vi "Arm Controller.vi"(8 "error in":errorcluster) -> ()   [LabVIEW 2018]
doc: "This VI executes continuously carrying out the current operation and responding to updates or new operations. It will often contain the timing or control code that is difficult to place directly in TeleOp. This VI generally opens all sensors and motors and isolates the rest of the robot code from knowing how the operations are carried out."
uses:
  <vilib>/Rock Robotics/WPI/Framework/Completion Status.ctl
  Arm Setpoints.ctl
  Arm Operations.ctl
  Arm Positions.ctl
  <vilib>/Rock Robotics/WPI/ThirdParty/Phoenix-LabVIEW/Motor Controller/Controls/CTRE_Phoenix_MotorControl_LimitSwitchSource_Local.ctl
  <vilib>/Rock Robotics/WPI/ThirdParty/Phoenix-LabVIEW/Motor Controller/Controls/CTRE_Phoenix_MotorControl_LimitSwitchNormal.ctl
  <vilib>/Rock Robotics/WPI/ThirdParty/Phoenix-LabVIEW/Motor Controller/Controls/CTRE_Phoenix_MotorControl_FeedbackDevice.ctl
  Turret Position.ctl
  <vilib>/Rock Robotics/WPI/ThirdParty/Phoenix-LabVIEW/Motor Controller/Controls/CTRE_Phoenix_MotorControl_ControlMode.ctl
  <vilib>/Rock Robotics/WPI/ThirdParty/Phoenix-LabVIEW/Motor Controller/Get/CTRE_Phoenix_MotorController_GetOutputCurrent_Enhanced.vi
  <vilib>/Rock Robotics/WPI/ThirdParty/Phoenix-LabVIEW/Motor Controller/Get/CTRE_Phoenix_MotorController_GetLimitSwitchStates.vi
  Arm Published Globals.vi
  Arm Constants.vi
  <vilib>/Rock Robotics/WPI/ThirdParty/Phoenix-LabVIEW/Motor Controller/Get/CTRE_Phoenix_MotorController_GetSelectedSensorData.vi
  <vilib>/Rock Robotics/Network Tables/NT Write Number.vi
  <vilib>/ptbypt/NI_PtbyPt.lvlib
  <vilib>/Rock Robotics/WPI/ThirdParty/Phoenix-LabVIEW/Controls/CTRE_Phoenix_Params.ctl
  <vilib>/Rock Robotics/Network Tables/NT Write Boolean.vi
panel:
  in  "P @ parallel to gnd elbow":dbl
  in  "P @ parallel to gnd":dbl
  in  "New Sensor Position 2":i32=-2
  in  "New Sensor Position":i32=-241
  in  "x":i32=500
  out "extensionLength":dbl=30.50305897767295
  out "wrist angle(deg)":dbl=27.45141836050927
  out "shoulder angle(deg)":dbl=92.24007561436673
  out "turret angle(deg)":dbl=45.049846153846154
  out "Theta4":dbl=207.45141836050928
  out "Theta3":dbl=36.40857303428192
  out "elbow angle(deg)":dbl=-51.35135135135135
  out "Position - Encoder Counts":T1(graph)={"Position (Raw Sensor Units)"=8134, "Position (Raw Sensor Units)"=-2127, "Position (Raw Sensor Units)"=-2299, "Position (Raw Sensor Units)"=1229}
  out "Position - Degrees":T2(graph)={"turret angle(deg)"=45.049846153846154, "shoulder angle(deg)"=92.24007561436673, "elbow angle(deg)"=-51.35135135135135, "wrist angle(deg)"=27.45141836050927}
  in  "Disable Logging":bool
  out "Current":T3(graph)
  in  "Interactive Values":T4
  out "Current\nCmd":string="Started at  22:56:16.335\nDefault: Reserve,  S 0.0, D 0.000000"
  in  "Buttons":cluster{"Execute Cmd":bool, "Abort Cmd":bool}
  out "Command Timing":cluster{"Start Time (ms)":u32, "Iterations":i32}={"Start Time (ms)"=8369965, "Iterations"=0}
  out "Status":T7
  # "Interactive Command: You may fill in the settings for a command\nand schedule it with the Execute button. You can observe and abort\nany command while fine tuning the code for the controller."
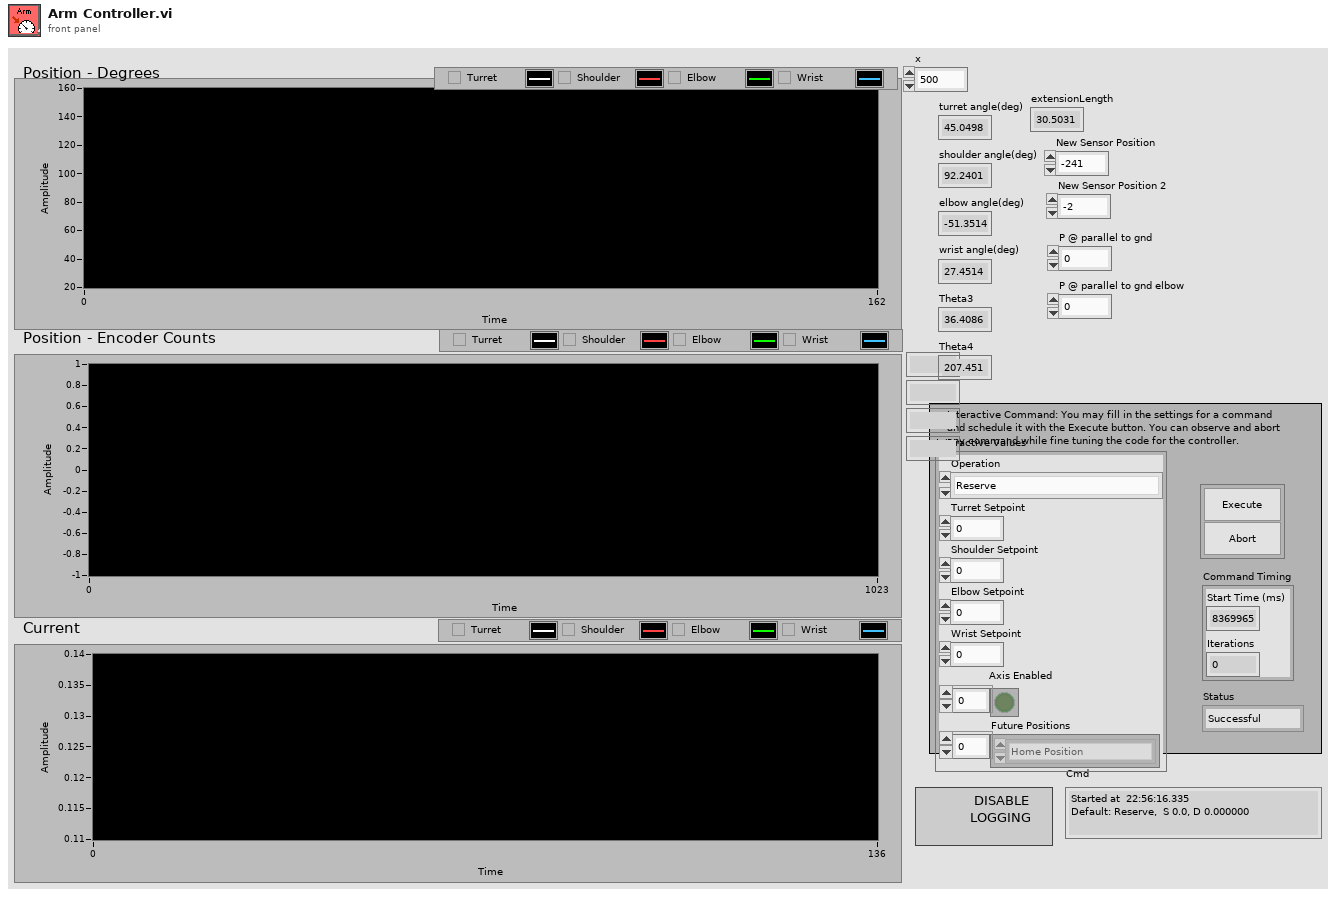
[diagram p1: front panel]
types:
  T1 = cluster{"Position (Raw Sensor Units)":i32, "Position (Raw Sensor Units)":i32, "Position (Raw Sensor Units)":i32, "Position (Raw Sensor Units)":i32}
  T2 = cluster{"turret angle(deg)":dbl, "shoulder angle(deg)":dbl, "elbow angle(deg)":dbl, "wrist angle(deg)":dbl}
  T3 = cluster{"Output Current":dbl, "Output Current":dbl, "Output Current":dbl, "Output Current":dbl}
  T4 = typedef "Arm Setpoints.ctl" = cluster{"Operation":T5, "Turret Setpoint":dbl, "Shoulder Setpoint":dbl, "Elbow Setpoint":dbl, "Wrist Setpoint":dbl, "Axis Enabled":bool[], "Future Positions":T6[]}
  T5 = typedef "Arm Operations.ctl" = enum16{"Reserve", "Read Current", "Immediate", "Move arm to position", "Reset Encoders", "Reset Turret", "Reset Shoulder", "Reset Elbow", "Reset Wrist", "Hold Encoder Counts"}
  T6 = typedef "Arm Positions.ctl" = enum16{"Home Position", "Safe Position", "Hatch - Ground", "Hatch - Low", "Hatch - Middle", "High - Safe", "Hatch - High", "Cargo - Low", "Cargo - Middle", "Cargo - High", "Cargo - Loading Station", "Hatch - Loading Station", "Cargo - Ground", "Turret - Left", "Turret - Front", "Turret - Right", "Turret - Back", "Climbing - Forward", "Middle - Safe", "Low - Safe", "Safe Elbow up"}
  T7 = typedef "Completion Status.ctl" = enum16{"Successful", "Aborted", "Incomplete"}
  T8 = typedef "CTRE_Phoenix_MotorControl_FeedbackDevice.ctl" = i8
  T9 = typedef "CTRE_Phoenix_MotorControl_LimitSwitchNormal.ctl" = enum16{"Normally Open", "Normally Closed", "Disabled"}
  T10 = typedef "CTRE_Phoenix_MotorControl_LimitSwitchSource_Local.ctl" = enum16{"Feedback Connector", "Remote Talon SRX", "Remote CANifier", "Deactivated"}
  T11 = typedef "CTRE_Phoenix_Params.ctl" = u16
  T12 = typedef "WPI_MotorControlDeviceRef.ctl" = cluster{"DeviceStatus":errorcluster, "Type":T13, "PWM":cluster{"PWM Channel":T14, "DeadBand":T15}, "CAN":cluster{"Device Number":u8, "SetOutput VI Ref":variant, "GetOutput VI Ref":variant, "Enable VI Ref":variant, "Disable VI Ref":variant, "Data":variant}, "Invert":bool, "DIO PWM":cluster{"PWM \"Enable\" Channel":T14, "DIOChannel":T16, "PWM Rate":dbl}}
  T13 = typedef "WPI_MotorControlType.ctl" = enum16{"PWM", "CAN", "DIO PWM"}
  T14 = typedef "FPGA_DIOPWMChannel.ctl" = enum8{"PWM 0", "PWM 1", "PWM 2", "PWM 3", "PWM 4", "PWM 5", "PWM 6", "PWM 7", "PWM 8", "PWM 9", "PWM MXP 0", "PWM MXP 1", "PWM MXP 2", "PWM MXP 3", "PWM MXP 4", "PWM MXP 5", "PWM MXP 6", "PWM MXP 7", "PWM MXP 8", "PWM MXP 9", "Invalid"}
  T15 = typedef "WPI_PWMDeadband.ctl" = cluster{"Name":string, "maxPositivePwm":i32, "minPositivePwm":i32, "centerPwm":i32, "maxNegativePwm":i32, "minNegativePwm":i32, "angularRange":u16}
  T16 = typedef "FPGA_DIOChannel.ctl" = enum8{"DIO 0", "DIO 1", "DIO 2", "DIO 3", "DIO 4", "DIO 5", "DIO 6", "DIO 7", "DIO 8", "DIO 9", "DIO MXP 0", "DIO MXP 1", "DIO MXP 2", "DIO MXP 3", "DIO MXP 4", "DIO MXP 5", "DIO MXP 6", "DIO MXP 7", "DIO MXP 8", "DIO MXP 9", "DIO MXP 10", "DIO MXP 11", "DIO MXP 12", "DIO MXP 13", "DIO MXP 14", "DIO MXP 15", "SPI Port CS1", "SPI Port CS2", "SPI Port CS3", "SPI Port MISO", "SPI Port MOSI", "Invalid"}
  T17 = typedef "Command Status Info.ctl" = cluster{"Name":string, "Status":T7, "notifier out":T18}
  T18 = typedef "Completion Notifier.ctl" = refnum<notifier>
  T19 = cluster{"Current Command":T4, "Command Timing":cluster{"Start Time (ms)":u32, "Iterations":i32}, "Command Arguments":cluster{"Command Info":T17, "Description":string, "Default Command":T4, "queue out":refnum<queue>, "Subsystem Name":string}}
  T20 = typedef "Turret Position.ctl" = enum16{"Back", "Left", "Front", "Right"}
  T21 = cluster{"Position (Raw Sensor Units)":i32, "Position (Raw Sensor Units)":i32, i32, i32}
  T22 = typedef "CTRE_Phoenix_MotorControl_ControlMode.ctl" = u16
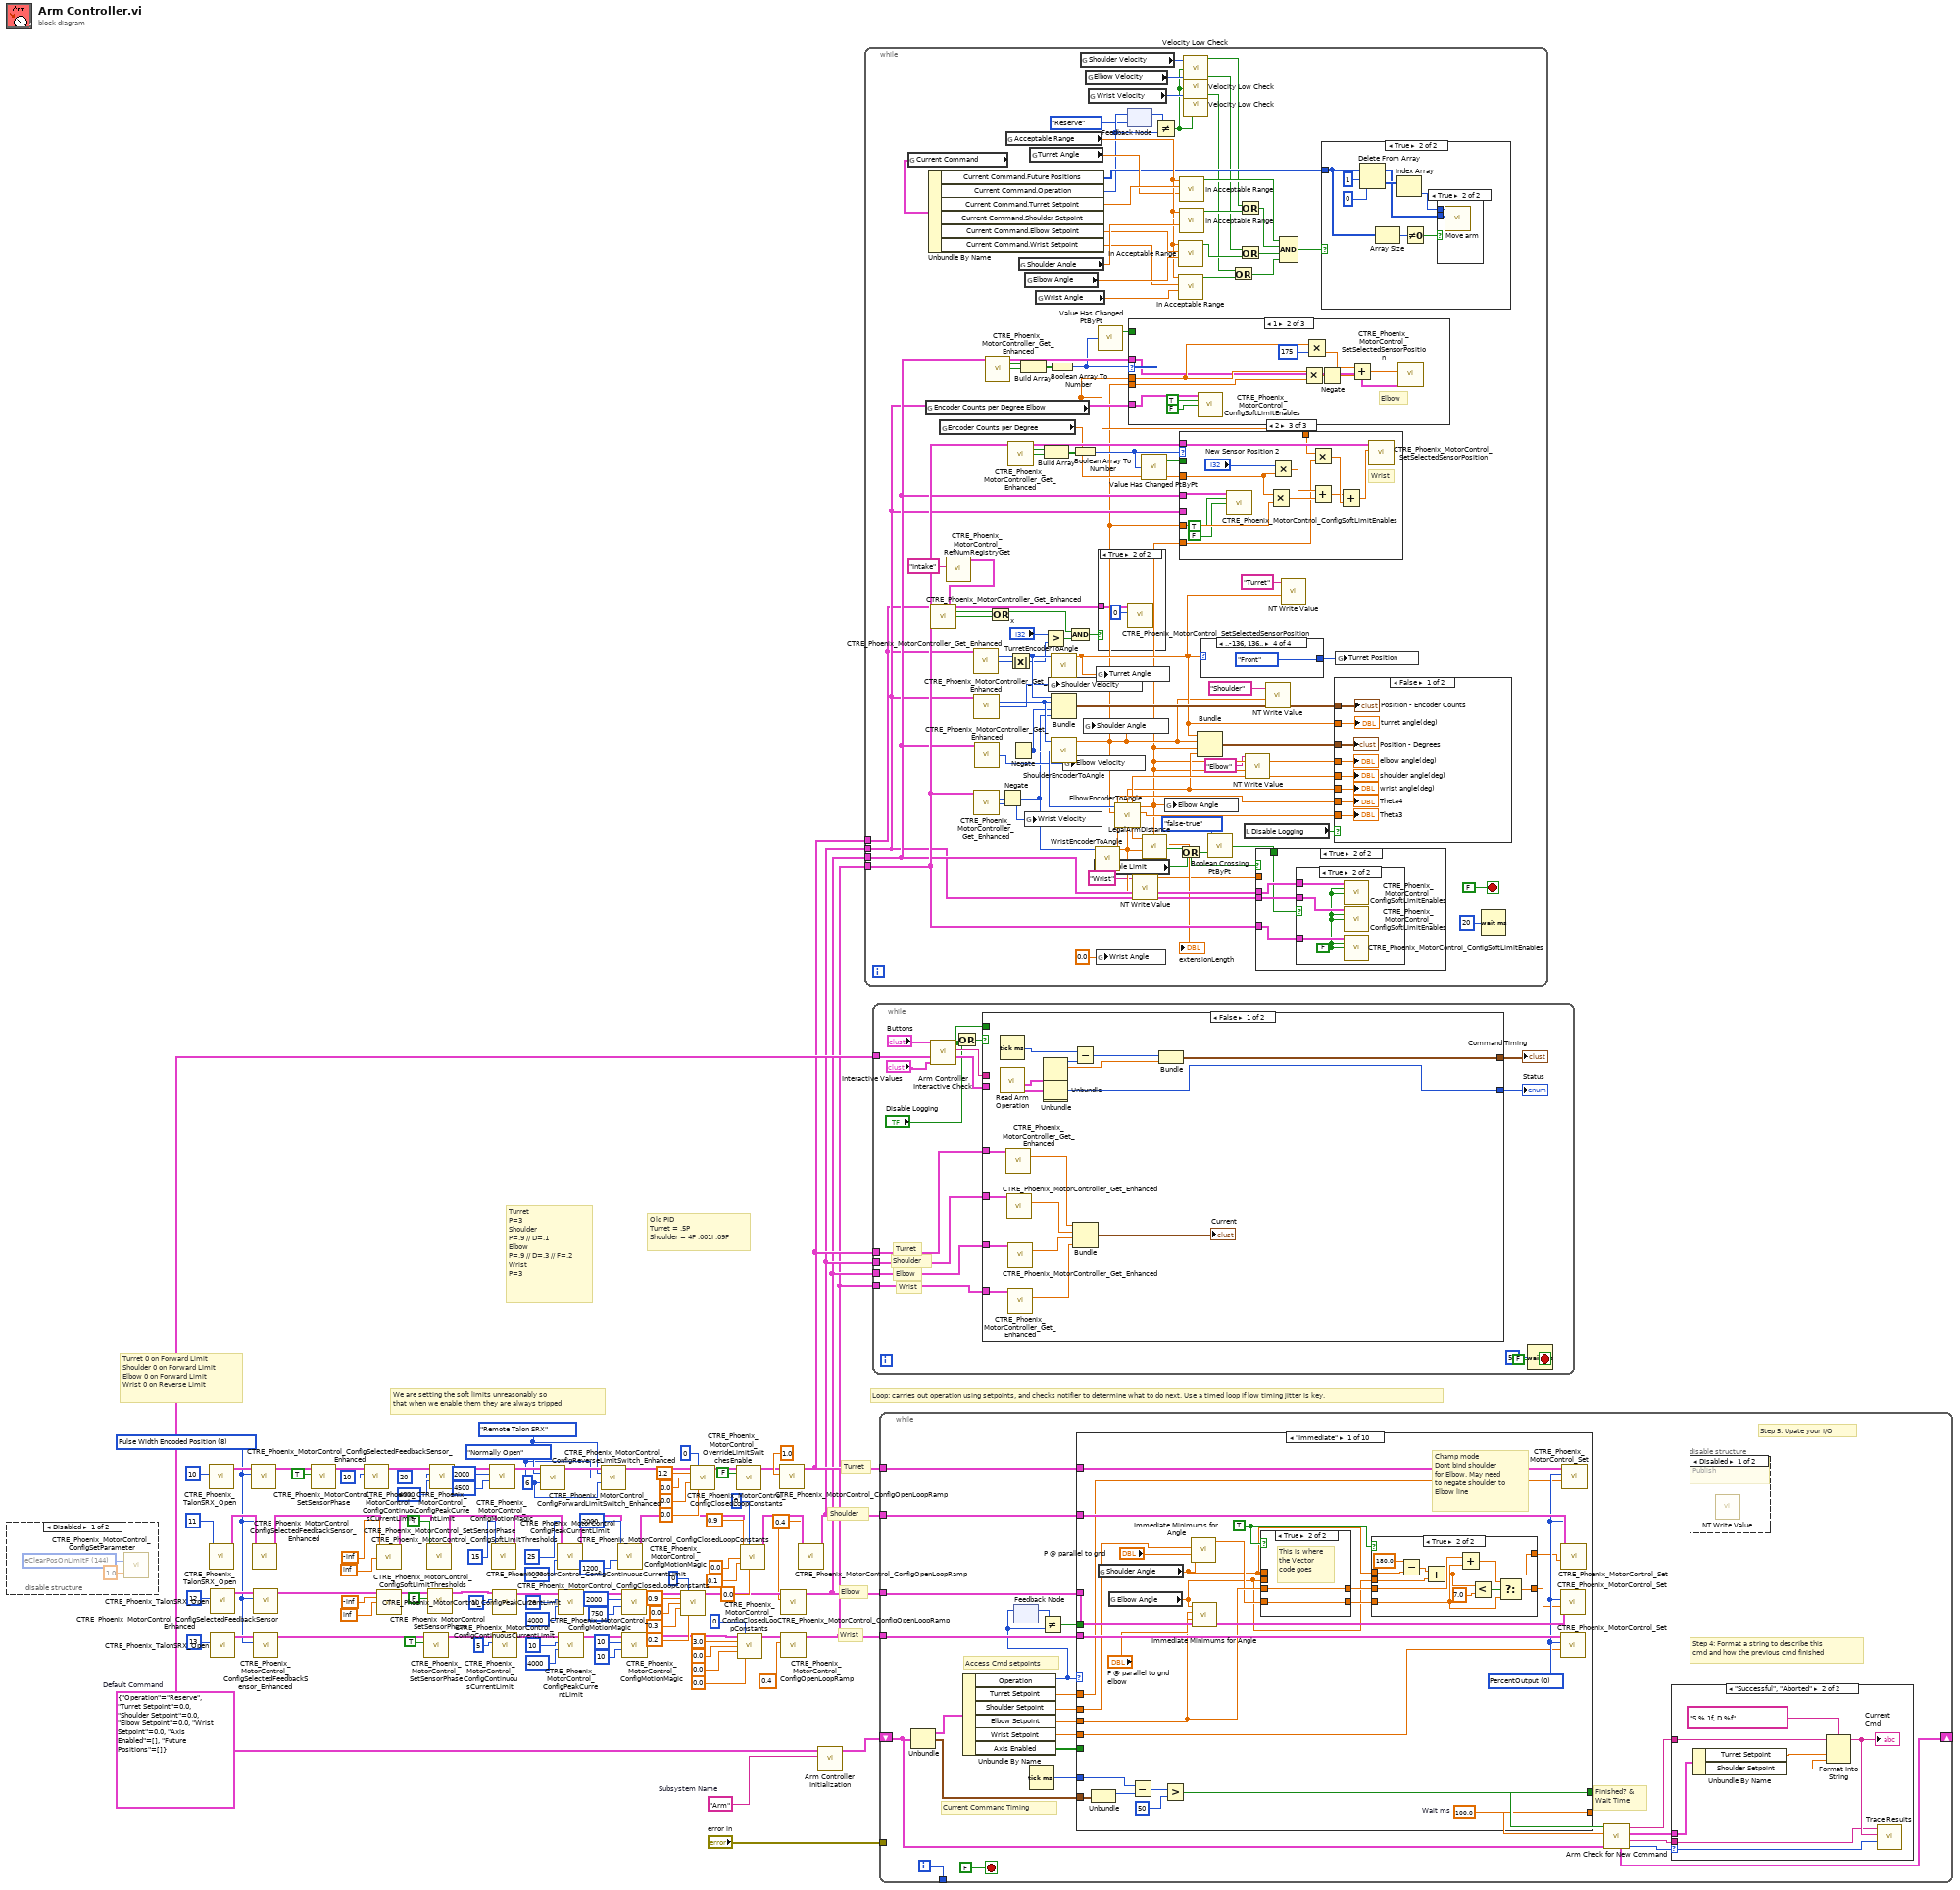
[diagram p0: block diagram]
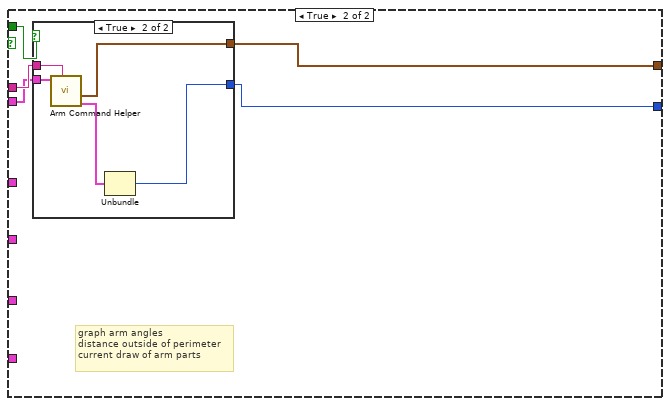
[diagram p3: hidden frame]
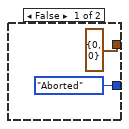
[diagram p4: hidden frame]
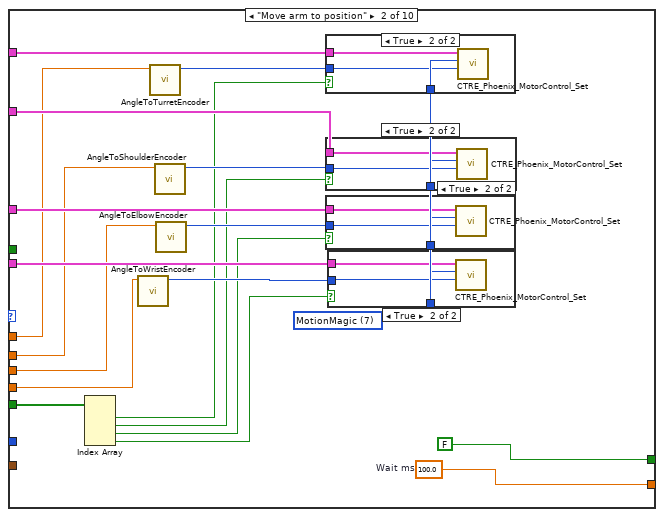
[diagram p9: hidden frame]
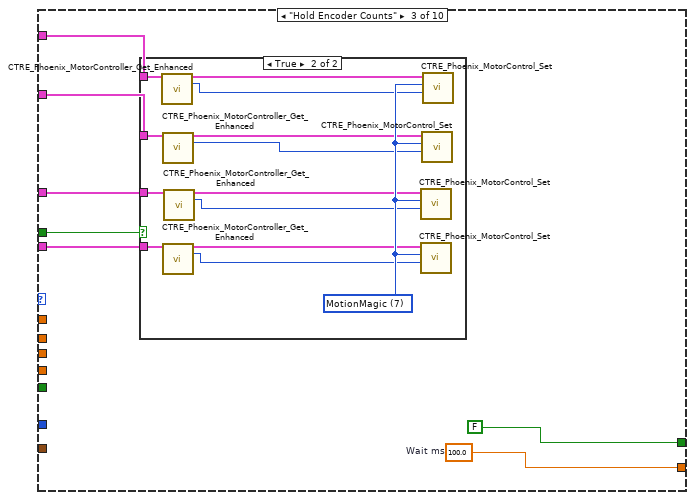
[diagram p14: hidden frame]
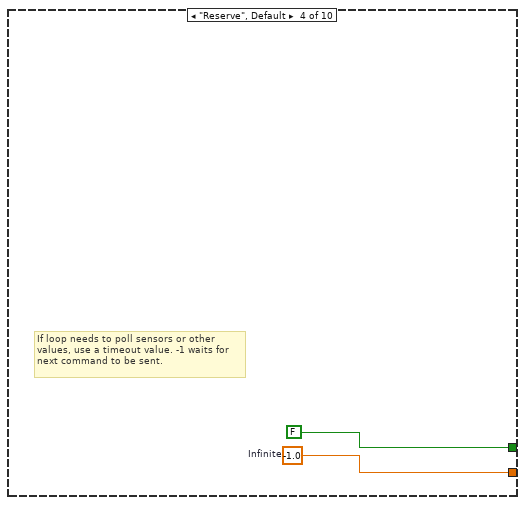
[diagram p16: hidden frame]
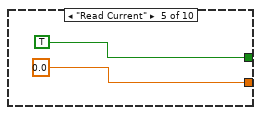
[diagram p17: hidden frame]
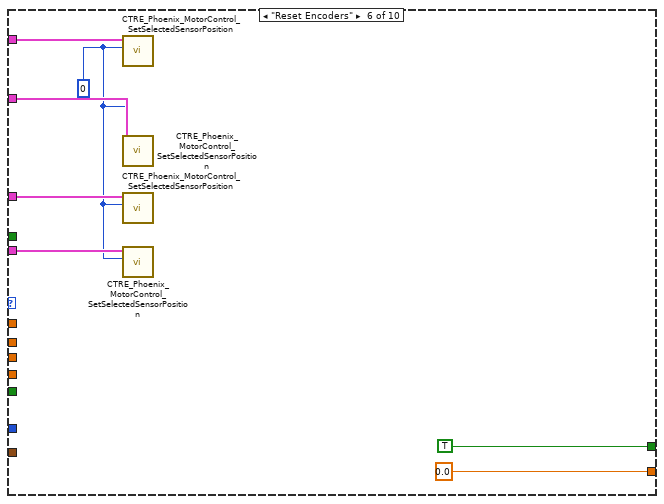
[diagram p18: hidden frame]
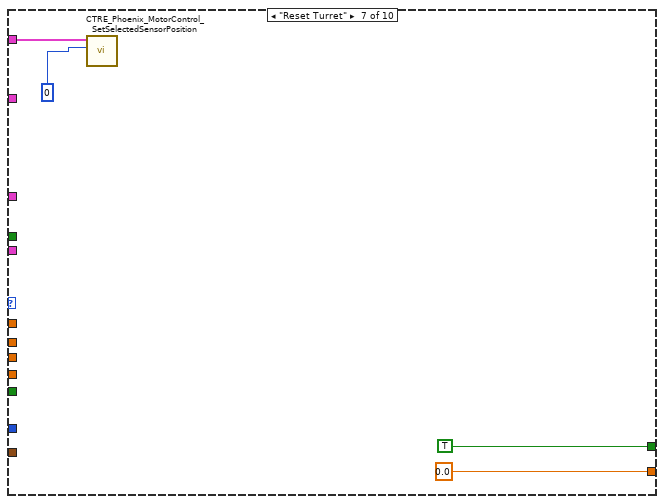
[diagram p19: hidden frame]
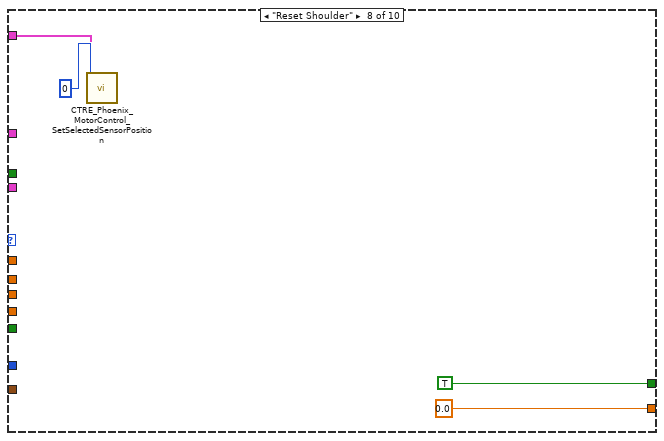
[diagram p20: hidden frame]
diagram:
  w2 = 0.4 ("secondsFromNeutralToFull")
  w3 = T8 8 items=["QuadEncoder"=0, "Analog"=2, "Tachometer"=4, "Pulse Width Encoded Position"=8, "Sensor Sum (S0 + S1)"=9, "Sensor Difference (D0 - D1)"=10, "Remote Source 0"=11, "Remote Source 1"=12, "Software Emulated"=15] ("Feedback Device")
  w37 = CTRE_Phoenix_MotorControl_LimitSwitchNormal."Normally Open" ("NormallyOpenOrClosed")
  w36 = 6 ("deviceID")
  w38 = CTRE_Phoenix_MotorControl_LimitSwitchSource_Local."Remote Talon SRX" ("Limit Switch Source")
  w98 = T4 {"Operation"=enum."Reserve", "Turret Setpoint"=0.0, "Shoulder Setpoint"=0.0, "Elbow Setpoint"=0.0, "Wrist Setpoint"=0.0, "Axis Enabled"=[], "Future Positions"=[]}  # Default Command
  w99 = "Arm"  # Subsystem Name
  # "We are setting the soft limits unreasonably so\nthat when we enable them they are always tripped"
  # "Turret 0 on Forward Limit\nShoulder 0 on Forward Limit\nElbow 0 on Forward Limit\nWrist 0 on Reverse Limit"
  # "Old PID\nTurret = .5P\nShoulder = 4P .001I .09F"
  # "Turret\nP=3\nShoulder\nP=.9 // D=.1\nElbow\nP=.9 // D=.3 // F=.2\nWrist\nP=3"
  # "Wrist"
  # "Elbow"
  # "Shoulder"
  # "Turret"
  # "Loop: carries out operation using setpoints, and checks notifier to determine what to do next. Use a timed loop if low timing jitter is key."
  n1 = disable-structure shown="Disabled" {
    frame Disabled {
      w103 = T11 144 items=["eOnBoot_BrakeMode"=31, "eQuadFilterEn"=91, "eQuadIdxPolarity"=108, "eClearPositionOnIdx"=100, "eMotionProfileHasUnderrunErr"=119, "eMotionProfileTrajectoryPointDurationMs"=120, "eClearPosOnLimitF"=144, "eClearPosOnLimitR"=145, "eStatusFramePeriod"=300, "eOpenLoopRamp"=301, "eClosedLoopRamp"=302, "eNeutralDeadband"=303, "ePeakPosOutput"=305, "eNominalPosOutput"=306, "ePeakNegOutput"=307, "eNominalNegOutput"=308, "eProfileParamSlot_P"=310, "eProfileParamSlot_I"=311, "eProfileParamSlot_D"=312, "eProfileParamSlot_F"=313, "eProfileParamSlot_IZone"=314, "eProfileParamSlot_AllowableErr"=315, "eProfileParamSlot_MaxIAccum"=316, "eProfileParamSlot_PeakOutput"=317, "eClearPositionOnLimitF"=320, "eClearPositionOnLimitR"=321, "eClearPositionOnQuadIdx"=322, "eSampleVelocityPeriod"=325, "eSampleVelocityWindow"=326, "eFeedbackSensorType"=330, "eSelectedSensorPosition"=331, "eFeedbackNotContinuous"=332, "eRemoteSensorSource"=333, "eRemoteSensorDeviceID"=334, "eSensorTerm"=335, "eRemoteSensorClosedLoopDisableNeutralOnLOS"=336, "ePIDLoopPolarity"=337, "ePIDLoopPeriod"=338, "eSelectedSensorCoefficient"=339, "eForwardSoftLimitThreshold"=340, "eReverseSoftLimitThreshold"=341, "eForwardSoftLimitEnable"=342, "eReverseSoftLimitEnable"=343, "eNominalBatteryVoltage"=350, "eBatterVoltageFilterSize"=351, "eContinuousCurrentLimitAmps"=360, "eContinuousCurrentLimitMs"=361, "ePeakCurrentLimitAmps"=362, "eClosedLoopIAccum"=370, "eCustomParam"=380, "eStickyFaults"=390, "eAnalogPosition"=400, "eQuadraturePosition"=401, "ePulseWidthPosition"=402, "eMotMag_Accel"=410, "eMotMag_VelCruise"=411, "eLimitSwitchSource"=421, "eLimitSwitchNormClosedAndDis"=422, "eLimitSwitchDisabledNeutralOnLOS"=423, "eLimitSwitchRemoteDevID"=424, "eSoftLimitDisabledNeutralOnLOS"=425, "ePulseWidthPeriod_EdgesPerRot"=430, "ePulseWidthPeriod_FilterWindowSz"=431] ("Parameter")
      n2 = call <vilib>:"CTRE_Phoenix_MotorControl_ConfigSetParameter.vi"("Parameter"=w103, "value"=1.0) -> ()  [unwired: 12 in, 2 out]
    }
    frame Enabled {
    }
  }
  n3 = call <vilib>:"CTRE_Phoenix_TalonSRX_Open.vi"("Device Number"=u8 10) -> ("CAN Talon SRX Ref"=w11:T12)  [unwired: 9 in, 1 out]
  n4 = call <vilib>:"CTRE_Phoenix_TalonSRX_Open.vi"("Device Number"=u8 11) -> ("CAN Talon SRX Ref"=w9:T12)  [unwired: 9 in, 1 out]
  n5 = call <vilib>:"CTRE_Phoenix_TalonSRX_Open.vi"("Device Number"=u8 12) -> ("CAN Talon SRX Ref"=w7:T12)  [unwired: 9 in, 1 out]
  n6 = call <vilib>:"CTRE_Phoenix_TalonSRX_Open.vi"("Device Number"=u8 13) -> ("CAN Talon SRX Ref"=w5:T12)  [unwired: 9 in, 1 out]
  n7 = call <vilib>:"CTRE_Phoenix_MotorControl_ConfigSelectedFeedbackSensor_Enhanced.vi"("Feedback Device"=w3, "PhoenixMotorControlDevRef"=w11) -> ("PhoenixMotorControlDevRef"=w10:T12)  [unwired: 8 in, 1 out]
  n8 = call <vilib>:"CTRE_Phoenix_MotorControl_ConfigSelectedFeedbackSensor_Enhanced.vi"("Feedback Device"=w3, "PhoenixMotorControlDevRef"=w9) -> ("PhoenixMotorControlDevRef"=w8:T12)  [unwired: 8 in, 1 out]
  n9 = call <vilib>:"CTRE_Phoenix_MotorControl_ConfigSelectedFeedbackSensor_Enhanced.vi"("Feedback Device"=w3, "PhoenixMotorControlDevRef"=w7) -> ("PhoenixMotorControlDevRef"=w6:T12)  [unwired: 8 in, 1 out]
  n10 = call <vilib>:"CTRE_Phoenix_MotorControl_ConfigSelectedFeedbackSensor_Enhanced.vi"("Feedback Device"=w3, "PhoenixMotorControlDevRef"=w5) -> ("PhoenixMotorControlDevRef"=w4:T12)  [unwired: 8 in, 1 out]
  n11 = call <vilib>:"CTRE_Phoenix_MotorControl_SetSensorPhase.vi"("PhaseSensor"=TRUE, "PhoenixMotorControlDevRef"=w10) -> ("PhoenixMotorControlDevRef"=w34:T12)  [unwired: 8 in, 1 out]
  n12 = call <vilib>:"CTRE_Phoenix_MotorControl_ConfigContinuousCurrentLimit.vi"("Continuous Current Limit (Amps)"=10, "PhoenixMotorControlDevRef"=w34) -> ("PhoenixMotorControlDevRef"=w83:T12)  [unwired: 8 in, 1 out]
  n13 = call <vilib>:"CTRE_Phoenix_MotorControl_ConfigSoftLimitThresholds.vi"("PhoenixMotorControlDevRef"=w8, "Forward Soft Limit"=-inf, "Reverse Soft Limit"=inf) -> ("PhoenixMotorControlDevRef"=w26:T12)  [unwired: 11 in, 1 out]
  n14 = call <vilib>:"CTRE_Phoenix_MotorControl_ConfigSoftLimitThresholds.vi"("PhoenixMotorControlDevRef"=w6, "Forward Soft Limit"=-inf, "Reverse Soft Limit"=inf) -> ("PhoenixMotorControlDevRef"=w21:T12)  [unwired: 11 in, 1 out]
  n15 = call <vilib>:"CTRE_Phoenix_MotorControl_SetSensorPhase.vi"("PhaseSensor"=TRUE, "PhoenixMotorControlDevRef"=w4) -> ("PhoenixMotorControlDevRef"=w29:T12)  [unwired: 8 in, 1 out]
  n16 = call <vilib>:"CTRE_Phoenix_MotorControl_SetSensorPhase.vi"("PhaseSensor"=TRUE, "PhoenixMotorControlDevRef"=w26) -> ("PhoenixMotorControlDevRef"=w27:T12)  [unwired: 8 in, 1 out]
  n17 = call <vilib>:"CTRE_Phoenix_MotorControl_SetSensorPhase.vi"("PhaseSensor"=FALSE, "PhoenixMotorControlDevRef"=w21) -> ("PhoenixMotorControlDevRef"=w28:T12)  [unwired: 8 in, 1 out]
  n18 = call <vilib>:"CTRE_Phoenix_MotorControl_ConfigPeakCurrentLimit.vi"("Peak Current Maximum Duration (ms)"=4000, "Peak Current (Amps)"=20, "PhoenixMotorControlDevRef"=w83) -> ("PhoenixMotorControlDevRef"=w66:T12)  [unwired: 7 in, 1 out]
  n19 = call <vilib>:"CTRE_Phoenix_MotorControl_ConfigMotionMagic.vi"("Acceleration"=4500, "Cruise Velocity"=2000, "PhoenixMotorControlDevRef"=w66) -> ("PhoenixMotorControlDevRef"=w41:T12)  [unwired: 7 in, 1 out]
  n20 = call <vilib>:"CTRE_Phoenix_MotorControl_ConfigContinuousCurrentLimit.vi"("Continuous Current Limit (Amps)"=15, "PhoenixMotorControlDevRef"=w27) -> ("PhoenixMotorControlDevRef"=w92:T12)  [unwired: 8 in, 1 out]
  n21 = call <vilib>:"CTRE_Phoenix_MotorControl_ConfigContinuousCurrentLimit.vi"("Continuous Current Limit (Amps)"=10, "PhoenixMotorControlDevRef"=w28) -> ("PhoenixMotorControlDevRef"=w93:T12)  [unwired: 8 in, 1 out]
  n22 = call <vilib>:"CTRE_Phoenix_MotorControl_ConfigContinuousCurrentLimit.vi"("Continuous Current Limit (Amps)"=5, "PhoenixMotorControlDevRef"=w29) -> ("PhoenixMotorControlDevRef"=w82:T12)  [unwired: 8 in, 1 out]
  n23 = call <vilib>:"CTRE_Phoenix_MotorControl_ConfigForwardLimitSwitch_Enhanced.vi"("PhoenixMotorControlDevRef"=w41, "Limit Switch Source"=w38, "NormallyOpenOrClosed"=w37, "deviceID"=w36) -> ("PhoenixMotorControlDevRef"=w40:T12)  [unwired: 10 in, 1 out]
  n24 = call <vilib>:"CTRE_Phoenix_MotorControl_ConfigPeakCurrentLimit.vi"("Peak Current Maximum Duration (ms)"=4000, "Peak Current (Amps)"=25, "PhoenixMotorControlDevRef"=w92) -> ("PhoenixMotorControlDevRef"=w69:T12)  [unwired: 7 in, 1 out]
  n25 = call <vilib>:"CTRE_Phoenix_MotorControl_ConfigPeakCurrentLimit.vi"("Peak Current Maximum Duration (ms)"=4000, "Peak Current (Amps)"=20, "PhoenixMotorControlDevRef"=w93) -> ("PhoenixMotorControlDevRef"=w72:T12)  [unwired: 7 in, 1 out]
  n26 = call <vilib>:"CTRE_Phoenix_MotorControl_ConfigPeakCurrentLimit.vi"("Peak Current Maximum Duration (ms)"=4000, "Peak Current (Amps)"=10, "PhoenixMotorControlDevRef"=w82) -> ("PhoenixMotorControlDevRef"=w77:T12)  [unwired: 7 in, 1 out]
  n27 = call <vilib>:"CTRE_Phoenix_MotorControl_ConfigReverseLimitSwitch_Enhanced.vi"("PhoenixMotorControlDevRef"=w40, "Limit Switch Source"=w38, "NormallyOpenOrClosed"=w37, "deviceID"=w36) -> ("PhoenixMotorControlDevRef"=w39:T12)  [unwired: 10 in, 1 out]
  n28 = call <vilib>:"CTRE_Phoenix_MotorControl_ConfigMotionMagic.vi"("Acceleration"=1200, "Cruise Velocity"=2000, "PhoenixMotorControlDevRef"=w69) -> ("PhoenixMotorControlDevRef"=w47:T12)  [unwired: 7 in, 1 out]
  n29 = call <vilib>:"CTRE_Phoenix_MotorControl_ConfigMotionMagic.vi"("Acceleration"=750, "Cruise Velocity"=2000, "PhoenixMotorControlDevRef"=w72) -> ("PhoenixMotorControlDevRef"=w48:T12)  [unwired: 7 in, 1 out]
  n30 = call <vilib>:"CTRE_Phoenix_MotorControl_ConfigMotionMagic.vi"("Acceleration"=10, "Cruise Velocity"=10, "PhoenixMotorControlDevRef"=w77) -> ("PhoenixMotorControlDevRef"=w49:T12)  [unwired: 7 in, 1 out]
  n31 = call <vilib>:"CTRE_Phoenix_MotorControl_ConfigClosedLoopConstants.vi"("PhoenixMotorControlDevRef"=w48, "slotIdx"=0, "P"=0.9, "I"=0.0, "D"=0.3 ("I"), "F"=0.2 ("I")) -> ("PhoenixMotorControlDevRef"=w15:T12)  [unwired: 8 in, 1 out]
  n32 = call <vilib>:"CTRE_Phoenix_MotorControl_ConfigClosedLoopConstants.vi"("PhoenixMotorControlDevRef"=w39, "slotIdx"=0, "P"=1.2, "I"=0.0, "D"=0.0 ("I"), "F"=0.0 ("I")) -> ("PhoenixMotorControlDevRef"=w42:T12)  [unwired: 8 in, 1 out]
  n33 = call <vilib>:"CTRE_Phoenix_MotorControl_OverrideLimitSwitchesEnable.vi"("PhoenixMotorControlDevRef"=w42, "Override Limit Switch Enable?"=FALSE) -> ("PhoenixMotorControlDevRef"=w19:T12)  [unwired: 12 in, 1 out]
  n34 = call <vilib>:"CTRE_Phoenix_MotorControl_ConfigClosedLoopConstants.vi"("PhoenixMotorControlDevRef"=w49, "slotIdx"=0, "P"=3.0, "I"=0.0, "D"=0.0 ("I"), "F"=0.0 ("I")) -> ("PhoenixMotorControlDevRef"=w13:T12)  [unwired: 8 in, 1 out]
  n35 = call <vilib>:"CTRE_Phoenix_MotorControl_ConfigClosedLoopConstants.vi"("PhoenixMotorControlDevRef"=w47, "slotIdx"=0, "P"=0.9, "I"=0.0, "D"=0.1 ("I"), "F"=0.0 ("I")) -> ("PhoenixMotorControlDevRef"=w17:T12)  [unwired: 8 in, 1 out]
  n36 = call <vilib>:"CTRE_Phoenix_MotorControl_ConfigOpenLoopRamp.vi"("secondsFromNeutralToFull"=1.0, "PhoenixMotorControlDevRef"=w19) -> ("PhoenixMotorControlDevRef"=w18:T12)  [unwired: 8 in, 1 out]
  n37 = call <vilib>:"CTRE_Phoenix_MotorControl_ConfigOpenLoopRamp.vi"("secondsFromNeutralToFull"=w2, "PhoenixMotorControlDevRef"=w15) -> ("PhoenixMotorControlDevRef"=w14:T12)  [unwired: 8 in, 1 out]
  n38 = call <vilib>:"CTRE_Phoenix_MotorControl_ConfigOpenLoopRamp.vi"("secondsFromNeutralToFull"=0.4, "PhoenixMotorControlDevRef"=w13) -> ("PhoenixMotorControlDevRef"=w12:T12)  [unwired: 8 in, 1 out]
  n39 = call <vilib>:"CTRE_Phoenix_MotorControl_ConfigOpenLoopRamp.vi"("secondsFromNeutralToFull"=w2, "PhoenixMotorControlDevRef"=w17) -> ("PhoenixMotorControlDevRef"=w16:T12)  [unwired: 8 in, 1 out]
  n40 = call "Arm Controller Initialization.vi"("Subsystem Name"=w99, "Default Command"=w98) -> ("Current Command"=w100:T19)  [unwired: 9 in]
  n41 = while {
    tunnel: w18 -> [w149]
    tunnel: w16 -> [w166]
    tunnel: w14 -> [w167]
    tunnel: w12 -> [w168]
    stop <- FALSE stop-if-true
    n42 = global read "Arm Published Globals.vi" "Current Command"() -> (w148:T19)
    n43 = global read "Arm Constants.vi" "Encoder Counts per Degree Elbow"() -> (w131:dbl)
    n44 = Unbundle By Name(w148) -> ("Current Command.Future Positions"=w134:T6[], "Current Command.Operation"=w117:T5, "Current Command.Turret Setpoint"=w141:dbl, "Current Command.Shoulder Setpoint"=w146:dbl, "Current Command.Elbow Setpoint"=w145:dbl, "Current Command.Wrist Setpoint"=w142:dbl)
    n45 = global read "Arm Constants.vi" "Encoder Counts per Degree"() -> (w176:dbl)
    n46 = call <vilib>:"CTRE_Phoenix_MotorControl_RefNumRegistryGet.vi"("refnum name"="Intake") -> ("PhoenixMotorControlDevRef"=w150:T12)  [unwired: 9 in, 1 out]
    n47 = call-poly <vilib>:"CTRE_Phoenix_MotorController_Get_Enhanced.vi"("PhoenixMotorControlDevRef"=w150) -> ("Forward Limit Closed?"=w155:bool, "Reverse Limit Closed?"=w152:bool)  [unwired: 11 in, 2 out]
    n48 = call-poly <vilib>:"CTRE_Phoenix_MotorController_Get_Enhanced.vi"("PhoenixMotorControlDevRef"=w149) -> ("Position (Raw Sensor Units)"=w190:i32, "Velocity (Raw Sensor Units per 100 ms)"=w159:i32)  [unwired: 11 in, 2 out]
    n49 = call-poly <vilib>:"CTRE_Phoenix_MotorController_Get_Enhanced.vi"("PhoenixMotorControlDevRef"=w166) -> ("Position (Raw Sensor Units)"=w191:i32, "Velocity (Raw Sensor Units per 100 ms)"=w130:i32)  [unwired: 11 in, 2 out]
    n50 = call-poly <vilib>:"CTRE_Phoenix_MotorController_Get_Enhanced.vi"("PhoenixMotorControlDevRef"=w168) -> ("Position (Raw Sensor Units)"=w187:i32, "Velocity (Raw Sensor Units per 100 ms)"=w128:i32)  [unwired: 11 in, 2 out]
    n51 = call-poly <vilib>:"CTRE_Phoenix_MotorController_Get_Enhanced.vi"("PhoenixMotorControlDevRef"=w167) -> ("Position (Raw Sensor Units)"=w162:i32, "Velocity (Raw Sensor Units per 100 ms)"=w129:i32)  [unwired: 11 in, 2 out]
    n52 = call-poly <vilib>:"CTRE_Phoenix_MotorController_Get_Enhanced.vi"("PhoenixMotorControlDevRef"=w167) -> ("PhoenixMotorControlDevRef"=w178:T12, "Forward Limit Closed?"=w185:bool, "Reverse Limit Closed?"=w184:bool)  [unwired: 11 in, 1 out]
    n53 = Or(x=w155, y=w152) -> (x .or. y?=w153:bool)
    n54 = Negate(x=w187) -> (-x=w122:i32)
    n55 = global read "Arm Constants.vi" "Acceptable Range"() -> (w140:dbl)
    n56 = call-poly <vilib>:"CTRE_Phoenix_MotorController_Get_Enhanced.vi"("PhoenixMotorControlDevRef"=w168) -> ("PhoenixMotorControlDevRef"=w177:T12, "Forward Limit Closed?"=w182:bool, "Reverse Limit Closed?"=w181:bool)  [unwired: 11 in, 1 out]
    n57 = Absolute Value(x=w159) -> (abs(x)=w154:i32)
    n58 = Negate(x=w162) -> (-x=w161:i32)
    n59 = global read "Arm Published Globals.vi" "Shoulder Angle"() -> (w147:dbl)
    n60 = Build Array(w185, w184) -> (w183:bool[])
    n61 = global write "Arm Published Globals.vi" "Wrist Velocity"(w128) -> ()
    n62 = global read "Arm Published Globals.vi" "Elbow Angle"() -> (w144:dbl)
    n63 = global read "Arm Published Globals.vi" "Turret Angle"() -> (w139:dbl)
    n64 = global read "Arm Published Globals.vi" "Wrist Angle"() -> (w143:dbl)
    n65 = Greater?(x="x", y=w154) -> (0:w158:bool)
    n66 = Build Array(w182, w181) -> (w180:bool[])
    n67 = global write "Arm Published Globals.vi" "Shoulder Velocity"(w130) -> ()
    n68 = Boolean Array To Number(Boolean array=w183) -> (number=w170:u32)
    n69 = call "TurretEncoderToAngle.vi"("encoderPulses"=w190) -> ("turret angle(deg)"=w113:dbl)  [unwired: 10 in]
    n70 = Bundle("Position (Raw Sensor Units)"=w190, "Position (Raw Sensor Units)"=w191, w161, w122) -> (w192:T21)  [unwired: 1 in]
    n71 = call "ShoulderEncoderToAngle.vi"("encoderPulses"=w191) -> ("shoulder angle(deg)"=w111:dbl)  [unwired: 9 in, 1 out]
    n72 = global write "Arm Published Globals.vi" "Elbow Velocity"(w129) -> ()
    n73 = And(x=w153, y=w158) -> (x .and. y?=w156:bool)
    n74 = Boolean Array To Number(Boolean array=w180) -> (number=w172:u32)
    n75 = global read "Arm Published Globals.vi" "Shoulder Velocity"() -> (w127:i32)
    n76 = global write "Arm Published Globals.vi" "Shoulder Angle"(w111) -> ()
    n77 = global read "Arm Published Globals.vi" "Elbow Velocity"() -> (w121:i32)
    n78 = global read "Arm Published Globals.vi" "Wrist Velocity"() -> (w119:i32)
    n79 = global read "Arm Published Globals.vi" "Disable Limit"() -> (w104:bool)
    n80 = call "WristEncoderToAngle.vi"("encoderPulses"=w122) -> ("Theta4"=w186:dbl, "wrist angle(deg)"=w109:dbl)  [unwired: 9 in]
    n81 = global write "Arm Published Globals.vi" "Turret Angle"(w113) -> ()
    n82 = global write "Arm Published Globals.vi" "Wrist Angle"(0.0 ("Wrist Angle")) -> ()
    n83 = call <vilib>:"Value Has Changed PtByPt.vi"("input data point"=w170) -> ("has changed"=w169:bool)  [unwired: 1 in, 1 out]
    n84 = case shown="True" w156 {
      tunnel: w149 -> [_ w223]
      frame False {
      }
      frame True {
        n85 = call <vilib>:"CTRE_Phoenix_MotorControl_SetSelectedSensorPosition.vi"("New Sensor Position"=0, "PhoenixMotorControlDevRef"=w223) -> ()  [unwired: 8 in, 2 out]
      }
    }
    n86 = call "ElbowEncoderToAngle.vi"("ElbowencoderPulses"=w161, "ShoulderAngle"=w111) -> ("elbow angle(deg)"=w107:dbl, "Theta3"=w179:dbl)  [unwired: 7 in]
    n87 = feedback-in #1(w117) -> ()
    n88 = feedback #1(Arm_Operations."Reserve" ("Operation")) -> (w116:T5)
    n89 = case shown="1" w170 {
      tunnel: w111 -> [_ w282 w293]
      tunnel: w131 -> [_ w279 w290]
      tunnel: w178 -> [_ w278 w289]
      tunnel: w166 -> [w271 w275 w288]
      tunnel: w169 -> [w270 _ _]
      frame 0, Default {
        n90 = First Call?() -> (First Call?: T/F=w268:bool)
        n91 = Or(x=w268, y=w270) -> (x .or. y?=w269:bool)
        n92 = case shown="True" w269 {
          tunnel: w271 -> [_ w273]
          frame False {
          }
          frame True {
            w272 = FALSE ("Reverse Soft Limit Enable")
            n93 = call <vilib>:"CTRE_Phoenix_MotorControl_ConfigSoftLimitEnables.vi"("PhoenixMotorControlDevRef"=w273, "Forward Soft Limit Enable"=w272, "Reverse Soft Limit Enable"=w272) -> ()  [unwired: 11 in, 2 out]
          }
        }
      }
      frame 1 {
        # "Elbow"
        n94 = call <vilib>:"CTRE_Phoenix_MotorControl_ConfigSoftLimitEnables.vi"("PhoenixMotorControlDevRef"=w275, "Forward Soft Limit Enable"=TRUE, "Reverse Soft Limit Enable"=FALSE) -> ()  [unwired: 11 in, 2 out]
        n95 = Multiply(x=w279, y=w282) -> (x*y=w281:dbl)
        n96 = Multiply(x=w279, y=175 ("New Sensor Position 2")) -> (x*y=w280:dbl)
        n97 = Negate(x=w281) -> (-x=w274:dbl)
        n98 = Add(x=w280, y=w274) -> (x+y=w283:dbl)
        n99 = call <vilib>:"CTRE_Phoenix_MotorControl_SetSelectedSensorPosition.vi"("New Sensor Position"=w283, "PhoenixMotorControlDevRef"=w278) -> ()  [unwired: 8 in, 2 out]
      }
      frame 2 {
        # "Elbow"
        n100 = call <vilib>:"CTRE_Phoenix_MotorControl_ConfigSoftLimitEnables.vi"("PhoenixMotorControlDevRef"=w288, "Forward Soft Limit Enable"=FALSE, "Reverse Soft Limit Enable"=TRUE) -> ()  [unwired: 11 in, 2 out]
        n101 = Multiply(x=w290, y=w293) -> (x*y=w292:dbl)
        n102 = Multiply(x=w290, y=-3 ("New Sensor Position")) -> (x*y=w291:dbl)
        n103 = Negate(x=w292) -> (-x=w285:dbl)
        n104 = Add(x=w291, y=w285) -> (x+y=w294:dbl)
        n105 = call <vilib>:"CTRE_Phoenix_MotorControl_SetSelectedSensorPosition.vi"("New Sensor Position"=w294, "PhoenixMotorControlDevRef"=w289) -> ()  [unwired: 8 in, 2 out]
      }
    }
    n106 = call-poly <vilib>:"NT Write Value.vi"("Numeric"=w109, "Name"="Wrist") -> ()  [unwired: 9 in, 1 out]
    n107 = call <vilib>:"Value Has Changed PtByPt.vi"("input data point"=w172) -> ("has changed"=w171:bool)  [unwired: 1 in, 1 out]
    n108 = call "LegalArmDistance.vi"("WristAngle"=w109, "ElbowAngle"=w107, "ShoulderAngle"=w111) -> ("extensionLength"=→"extensionLength":dbl, "isBelowThirty"=w165:bool)  [unwired: 7 in]
    n109 = Not Equal?(x=w116, y=w117) -> (x != y?=w114:bool)
    n110 = global write "Arm Published Globals.vi" "Elbow Angle"(w107) -> ()
    n111 = call "In Acceptable Range.vi"("Variable"=w144, "Setpoint"=w145, "Acceptable Range"=w140) -> ("Boolean"=w136:bool)  [unwired: 8 in]
    n112 = call "In Acceptable Range.vi"("Variable"=w143, "Setpoint"=w142, "Acceptable Range"=w140) -> ("Boolean"=w135:bool)  [unwired: 8 in]
    n113 = Or(x=w165, y=w104) -> (x .or. y?=w105:bool)
    n114 = call "In Acceptable Range.vi"("Variable"=w139, "Setpoint"=w141, "Acceptable Range"=w140) -> ("Boolean"=w138:bool)  [unwired: 8 in]
    n115 = call "In Acceptable Range.vi"("Variable"=w147, "Setpoint"=w146, "Acceptable Range"=w140) -> ("Boolean"=w137:bool)  [unwired: 8 in]
    n116 = case shown="2" w172 {
      tunnel: w111 -> [_ w251 w265]
      tunnel: w176 -> [_ w249 w263]
      tunnel: w107 -> [_ w248 w262]
      tunnel: w177 -> [_ w244 w258]
      tunnel: w167 -> [w236 w243 w255]
      tunnel: w166 -> [w234 _ _]
      tunnel: w171 -> [w235 _ _]
      tunnel: w131 -> [_ w240 w254]
      frame 0, Default {
        n117 = First Call?() -> (First Call?: T/F=w232:bool)
        n118 = Or(x=w235, y=w232) -> (x .or. y?=w233:bool)
        n119 = case shown="True" w233 {
          tunnel: w236 -> [_ w239]
          tunnel: w234 -> [_ w238]
          frame False {
          }
          frame True {
            w237 = FALSE ("Forward Soft Limit Enable")
            n120 = call <vilib>:"CTRE_Phoenix_MotorControl_ConfigSoftLimitEnables.vi"("PhoenixMotorControlDevRef"=w239, "Forward Soft Limit Enable"=w237, "Reverse Soft Limit Enable"=w237) -> ()  [unwired: 11 in, 2 out]
            n121 = call <vilib>:"CTRE_Phoenix_MotorControl_ConfigSoftLimitEnables.vi"("PhoenixMotorControlDevRef"=w238, "Forward Soft Limit Enable"=w237, "Reverse Soft Limit Enable"=w237) -> ()  [unwired: 11 in, 2 out]
          }
        }
      }
      frame 1 {
        # "Wrist"
        n122 = call <vilib>:"CTRE_Phoenix_MotorControl_ConfigSoftLimitEnables.vi"("PhoenixMotorControlDevRef"=w243, "Forward Soft Limit Enable"=FALSE, "Reverse Soft Limit Enable"=TRUE) -> ()  [unwired: 11 in, 2 out]
        n123 = Multiply(x="New Sensor Position", y=w249) -> (x*y=w253:dbl)
        n124 = Multiply(x=w249, y=w251) -> (x*y=w252:dbl)
        n125 = Multiply(x=w240, y=w248) -> (x*y=w247:dbl)
        n126 = Add(x=w253, y=w252) -> (x+y=w246:dbl)
        n127 = Add(x=w246, y=w247) -> (x+y=w245:dbl)
        n128 = call <vilib>:"CTRE_Phoenix_MotorControl_SetSelectedSensorPosition.vi"("New Sensor Position"=w245, "PhoenixMotorControlDevRef"=w244) -> ()  [unwired: 8 in, 2 out]
      }
      frame 2 {
        # "Wrist"
        n129 = call <vilib>:"CTRE_Phoenix_MotorControl_ConfigSoftLimitEnables.vi"("PhoenixMotorControlDevRef"=w255, "Forward Soft Limit Enable"=TRUE, "Reverse Soft Limit Enable"=FALSE) -> ()  [unwired: 11 in, 2 out]
        n130 = Multiply(x=w263, y=w265) -> (x*y=w266:dbl)
        n131 = Multiply(x="New Sensor Position 2", y=w263) -> (x*y=w267:dbl)
        n132 = Multiply(x=w254, y=w262) -> (x*y=w261:dbl)
        n133 = Add(x=w267, y=w266) -> (x+y=w260:dbl)
        n134 = Add(x=w260, y=w261) -> (x+y=w259:dbl)
        n135 = call <vilib>:"CTRE_Phoenix_MotorControl_SetSelectedSensorPosition.vi"("New Sensor Position"=w259, "PhoenixMotorControlDevRef"=w258) -> ()  [unwired: 8 in, 2 out]
      }
    }
    n136 = call "Velocity Low Check.vi"("Initialize"=w114, "Shoulder Velocity"=w127) -> ("Velocity Low for Time"=w125:bool)  [unwired: 9 in]
    n137 = call "Velocity Low Check.vi"("Initialize"=w114, "Shoulder Velocity"=w121) -> ("Velocity Low for Time"=w120:bool)  [unwired: 9 in]
    n138 = call "Velocity Low Check.vi"("Initialize"=w114, "Shoulder Velocity"=w119) -> ("Velocity Low for Time"=w118:bool)  [unwired: 9 in]
    n139 = Bundle("turret angle(deg)"=w113, "shoulder angle(deg)"=w111, "elbow angle(deg)"=w107, "wrist angle(deg)"=w109) -> (w189:T2)  [unwired: 1 in]
    n140 = case shown="..-136, 136.." w113 {
      tunnel: [Turret_Position."Back" ("Turret Position") Turret_Position."Left" ("Turret Position") Turret_Position."Right" ("Turret Position") Turret_Position."Front" ("Turret Position")] -> w188
      frame -45..45 {
      }
      frame -135..-46 {
      }
      frame 46..135 {
      }
      frame ..-136, 136.. {
      }
    }
    n141 = call <vilib>:"Boolean Crossing PtByPt.vi"("direction"=enum16{"either", "false-true", "true-false"}."false-true", "input"=w105) -> ("crossing"=w163:bool)  [unwired: 1 in]
    n142 = Or(x=w118, y=w135) -> (x .or. y?=w123:bool)
    n143 = Or(x=w125, y=w137) -> (x .or. y?=w126:bool)
    n144 = Or(x=w120, y=w136) -> (x .or. y?=w124:bool)
    n145 = local read "Disable Logging"() -> (w173:bool)
    n146 = call-poly <vilib>:"NT Write Value.vi"("Numeric"=w107, "Name"="Elbow") -> ()  [unwired: 9 in, 1 out]
    n147 = case shown="True" w105 {
      tunnel: w107 -> [w200 _]
      tunnel: w168 -> [w197 w205]
      tunnel: w167 -> [w196 w207]
      tunnel: w166 -> [w195 w206]
      tunnel: w163 -> [_ w204]
      frame False {
        w193 = TRUE ("Forward Soft Limit Enable")
        w194 = FALSE ("Forward Soft Limit Enable")
        n148 = Greater Or Equal To 0?(x=w200) -> (x >= 0?=w199:bool)
        n149 = Not(x=w199) -> (.not. x?=w198:bool)
        n150 = call <vilib>:"CTRE_Phoenix_MotorControl_ConfigSoftLimitEnables.vi"("PhoenixMotorControlDevRef"=w196, "Forward Soft Limit Enable"=w199, "Reverse Soft Limit Enable"=w198) -> ()  [unwired: 11 in, 2 out]
        n151 = call <vilib>:"CTRE_Phoenix_MotorControl_ConfigSoftLimitEnables.vi"("PhoenixMotorControlDevRef"=w195, "Forward Soft Limit Enable"=w194, "Reverse Soft Limit Enable"=w193) -> ()  [unwired: 11 in, 2 out]
        n152 = disable-structure shown="Disabled" {
          disable-tunnel: w197 -> [w203 _]
          disable-tunnel: w194 -> [w202 _]
          disable-tunnel: w193 -> [w201 _]
          frame Disabled {
            n153 = call <vilib>:"CTRE_Phoenix_MotorControl_ConfigSoftLimitEnables.vi"("PhoenixMotorControlDevRef"=w203, "Forward Soft Limit Enable"=w202, "Reverse Soft Limit Enable"=w201) -> ()  [unwired: 11 in, 2 out]
          }
          frame Enabled {
          }
        }
      }
      frame True {
        n154 = case shown="True" w204 {
          tunnel: w207 -> [_ w211]
          tunnel: w206 -> [_ w210]
          tunnel: w205 -> [_ w209]
          frame False {
          }
          frame True {
            w208 = FALSE ("Reverse Soft Limit Enable")
            n155 = call <vilib>:"CTRE_Phoenix_MotorControl_ConfigSoftLimitEnables.vi"("PhoenixMotorControlDevRef"=w211, "Forward Soft Limit Enable"=w208, "Reverse Soft Limit Enable"=w208) -> ()  [unwired: 11 in, 2 out]
            n156 = call <vilib>:"CTRE_Phoenix_MotorControl_ConfigSoftLimitEnables.vi"("PhoenixMotorControlDevRef"=w210, "Forward Soft Limit Enable"=w208, "Reverse Soft Limit Enable"=w208) -> ()  [unwired: 11 in, 2 out]
            n157 = call <vilib>:"CTRE_Phoenix_MotorControl_ConfigSoftLimitEnables.vi"("PhoenixMotorControlDevRef"=w209, "Forward Soft Limit Enable"=w208, "Reverse Soft Limit Enable"=w208) -> ()  [unwired: 11 in, 2 out]
          }
        }
      }
    }
    n158 = call-poly <vilib>:"NT Write Value.vi"("Numeric"=w111, "Name"="Shoulder") -> ()  [unwired: 9 in, 1 out]
    n159 = Compound Arithmetic op=AND(w138, w126, w124, w123) -> (w133:bool)
    n160 = call-poly <vilib>:"NT Write Value.vi"("Numeric"=w113, "Name"="Turret") -> ()  [unwired: 9 in, 1 out]
    n161 = case shown="True" w133 {
      tunnel: w134 -> [_ w213]
      frame False {
      }
      frame True {
        n162 = Delete From Array(array=w213, length=1, index=0) -> (deleted portion=w217:T6[], array with subset deleted=w215:T6[])
        n163 = Array Size(array=w213) -> (size(s)=w214:i32)
        n164 = Index Array(array=w217) -> (element=w216:T6)  [unwired: 1 in]
        n165 = Not Equal To 0?(x=w214) -> (x != 0?=w212:bool)
        n166 = case shown="True" w212 {
          tunnel: w216 -> [_ w221]
          tunnel: w215 -> [_ w220]
          frame False {
          }
          frame True {
            n167 = call "Move arm.vi"("Future Positions"=w220, "Arm Position"=w221) -> ()  [unwired: 9 in, 1 out]
          }
        }
      }
    }
    n168 = case shown="False" w173 {
      tunnel: w192 -> [w231 _]
      tunnel: w189 -> [w230 _]
      tunnel: w113 -> [w229 _]
      tunnel: w186 -> [w228 _]
      tunnel: w111 -> [w227 _]
      tunnel: w107 -> [w226 _]
      tunnel: w109 -> [w225 _]
      tunnel: w179 -> [w224 _]
      frame False {
        "Position - Degrees" <- w230
        "Position - Encoder Counts" <- w231
        "elbow angle(deg)" <- w226
        "Theta3" <- w224
        "Theta4" <- w228
        "turret angle(deg)" <- w229
        "shoulder angle(deg)" <- w227
        "wrist angle(deg)" <- w225
      }
      frame True {
      }
    }
    n169 = global write "Arm Published Globals.vi" "Turret Position"(w188) -> ()
    n170 = Wait (ms)(milliseconds to wait=u32 20) -> ()  [unwired: 1 out]
  }
  n171 = while {
    tunnel: w98 -> [w312]
    tunnel: w18 -> [w306]
    tunnel: w16 -> [w305]
    tunnel: w14 -> [w301]
    tunnel: w12 -> [w300]
    stop <- FALSE stop-if-true
    # "Wrist"
    # "Elbow"
    # "Shoulder"
    # "Turret"
    n172 = call "Arm Controller Interactive Check.vi"("Interactive Command in"="Interactive Values", "Default Command"=w312, "Buttons"="Buttons") -> ("Interactive Command out"=w310:T4, "Trace String"=w311:string, "Schedule"=w302:bool)  [unwired: 6 in]
    n173 = Or(x="Disable Logging", y=w302) -> (x .or. y?=w304:bool)
    n174 = case shown="False" w304 {
      tunnel: [w332 w337] -> w309
      tunnel: w310 -> [_ w335]
      tunnel: [w328 w334] -> w308
      tunnel: w311 -> [_ w336]
      tunnel: w306 -> [w324 _]
      tunnel: w305 -> [w323 _]
      tunnel: w301 -> [w322 _]
      tunnel: w300 -> [w321 _]
      tunnel: w302 -> [_ w333]
      frame False {
        n175 = Tick Count (ms)() -> (millisecond timer value=w327:u32)
        n176 = call "Read Arm Operation.vi"() -> ("Command Info"=w325:T17, "SubSystem Data"=w326:T4)  [unwired: 9 in, 1 out]
        n177 = call-poly <vilib>:"CTRE_Phoenix_MotorController_Get_Enhanced.vi"("PhoenixMotorControlDevRef"=w324) -> ("Output Current"=w320:dbl)  [unwired: 12 in, 2 out]
        n178 = call-poly <vilib>:"CTRE_Phoenix_MotorController_Get_Enhanced.vi"("PhoenixMotorControlDevRef"=w323) -> ("Output Current"=w319:dbl)  [unwired: 12 in, 2 out]
        n179 = call-poly <vilib>:"CTRE_Phoenix_MotorController_Get_Enhanced.vi"("PhoenixMotorControlDevRef"=w322) -> ("Output Current"=w318:dbl)  [unwired: 12 in, 2 out]
        n180 = call-poly <vilib>:"CTRE_Phoenix_MotorController_Get_Enhanced.vi"("PhoenixMotorControlDevRef"=w321) -> ("Output Current"=w317:dbl)  [unwired: 12 in, 2 out]
        n181 = Unbundle(w326) -> ("Operation"=w331:T5, "Turret Setpoint"=w329:dbl)  [unwired: 5 out]
        n182 = Unbundle(w325) -> ("Status"=w332:T7)  [unwired: 2 out]
        n183 = Subtract(x=w327, y=w331) -> (x-y=w330:u32)
        n184 = Bundle("Output Current"=w320, "Output Current"=w319, "Output Current"=w318, "Output Current"=w317) -> (→"Current":T3)  [unwired: 1 in]
        n185 = Bundle(w330, "Turret Setpoint"=w329) -> (w328:cluster{u32, "Turret Setpoint":dbl})  [unwired: 1 in]
      }
      frame True {
        # "graph arm angles\ndistance outside of perimeter\ncurrent draw of arm parts"
        n186 = case shown="True" w333 {
          tunnel: [Completion_Status."Aborted" ("Status") w344] -> w337
          tunnel: w336 -> [_ w343]
          tunnel: w335 -> [_ w342]
          tunnel: [cluster{"Start Time (ms)":u32, "Iterations":i32} {"Start Time (ms)"=0, "Iterations"=0} ("Command Timing") w340] -> w334
          frame False {
          }
          frame True {
            n187 = call "Arm Command Helper.vi"("Description"=w343, "SubSystem Data"=w342) -> ("Command Info Out"=w341:T17, "Command Timing"=w340:cluster{"Start Time (ms)":u32, "Iterations":i32})  [unwired: 7 in, 1 out]
            n188 = Unbundle(w341) -> ("Status"=w344:T7)  [unwired: 2 out]
          }
        }
      }
    }
    "Status" <- w309
    "Command Timing" <- w308
    n189 = Wait (ms)(milliseconds to wait=u32 50) -> ()  [unwired: 1 out]
  }
  n190 = while {
    shift-right: [w362] -> _
    shift-left: w100 -> [w355]
    tunnel: [w368] -> _
    tunnel: "error in" -> [_]
    tunnel: w18 -> [w354]
    tunnel: w16 -> [w353]
    tunnel: w14 -> [w352]
    tunnel: w12 -> [w351]
    i -> [w368]
    stop <- FALSE stop-if-true
    # "Step 5: Upate your I/O"
    # "Step 4: Format a string to describe this\ncmd and how the previous cmd finished"
    # "Current Command Timing"
    # "Access Cmd setpoints"
    # "Finished? &\nWait Time"
    n191 = Unbundle(w355) -> ("Current Command"=w367:T4, "Command Timing"=w364:cluster{"Start Time (ms)":u32, "Iterations":i32})  [unwired: 1 out]
    n192 = Unbundle By Name(w367) -> ("Operation"=w346:T5, "Turret Setpoint"=w366:dbl, "Shoulder Setpoint"=w363:dbl, "Elbow Setpoint"=w350:dbl, "Wrist Setpoint"=w349:dbl, "Axis Enabled"=w348:bool[])
    n193 = feedback #2() -> (w347:T5)  [unwired: 1 in]
    n194 = feedback-in #2(w346) -> ()
    n195 = Tick Count (ms)() -> (millisecond timer value=w365:u32)
    n196 = Not Equal?(x=w347, y=w346) -> (x != y?=w345:bool)
    n197 = case shown="\"Immediate\"" w346 {
      tunnel: [w403 w440 w459 w474 0.0 ("Infinite") 0.0 ("Infinite") 0.0 ("Infinite") 0.0 ("Infinite") 0.0 ("Infinite") 0.0 ("Infinite")] -> w360
      tunnel: [w397 FALSE ("ignore previous (F)") FALSE ("ignore previous (F)") FALSE ("ignore previous (F)") TRUE ("ignore previous (F)") TRUE ("ignore previous (F)") TRUE ("ignore previous (F)") TRUE ("ignore previous (F)") TRUE ("ignore previous (F)") TRUE ("ignore previous (F)")] -> w361
      tunnel: w364 -> [w399 _ _ _ _ _ _ _ _ _]
      tunnel: w366 -> [w390 w429 _ _ _ _ _ _ _ _]
      tunnel: w365 -> [w398 _ _ _ _ _ _ _ _ _]
      tunnel: w363 -> [w387 w428 _ _ _ _ _ _ _ _]
      tunnel: w354 -> [w391 w436 w457 _ _ w483 w486 _ _ _]
      tunnel: w353 -> [w396 w439 w456 _ _ w480 _ w490 _ _]
      tunnel: w352 -> [w395 w435 w455 _ _ w481 _ _ w494 _]
      tunnel: w351 -> [w394 w438 w454 _ _ w482 _ _ _ w498]
      tunnel: w350 -> [w384 w427 _ _ _ _ _ _ _ _]
      tunnel: w349 -> [w392 w426 _ _ _ _ _ _ _ _]
      tunnel: w348 -> [_ w425 _ _ _ _ _ _ _ _]
      tunnel: w345 -> [_ _ w453 _ _ _ _ _ _ _]
      frame "Immediate" {
        w380 = TRUE
        w393 = T22 0 items=["PercentOutput"=0, "Position"=1, "Velocity"=2, "Current"=3, "Follower"=5, "MotionProfile"=6, "MotionMagic"=7, "MotionProfileArc"=10, "Disabled"=15] ("Control Mode")
        w403 = 100.0  # Wait ms
        # "This is where\nthe Vector \ncode goes"
        # "Champ mode\nDont bind shoulder\nfor Elbow. May need \nto negate shoulder to \nElbow line"
        n198 = Unbundle(w399) -> ("Start Time (ms)"=w402:u32)  [unwired: 1 out]
        n199 = global read "Arm Published Globals.vi" "Shoulder Angle"() -> (w379:dbl)
        n200 = global read "Arm Published Globals.vi" "Elbow Angle"() -> (w378:dbl)
        n201 = Subtract(x=w398, y=w402) -> (x-y=w401:u32)
        n202 = Greater?(x=w401, y=u8 50 ("Left Motor")) -> (0:w397:bool)
        n203 = call "Immediate Minimums for Angle.vi"("Power @ parallel to ground"="P @ parallel to gnd", "Input"=w387, "Angle"=w379) -> ("Output"=w382:dbl)  [unwired: 8 in]
        n204 = call "Immediate Minimums for Angle.vi"("Power @ parallel to ground"="P @ parallel to gnd elbow", "Input"=w384, "Angle"=w378) -> ()  [unwired: 8 in, 1 out]
        n205 = case shown="True" w380 {
          tunnel: w379 -> [_ _]
          tunnel: w378 -> [_ _]
          tunnel: [w405 w407] -> w383
          tunnel: w384 -> [w405 w407]
          tunnel: [w404 w406] -> w381
          tunnel: w382 -> [w404 w406]
          frame False {
          }
          frame True {
          }
        }
        n206 = case shown="True" w380 {
          tunnel: [w409 w410] -> w386
          tunnel: w381 -> [w409 w418]
          tunnel: [w408 w415] -> w385
          tunnel: w383 -> [w408 w417]
          tunnel: w378 -> [_ w413]
          tunnel: w379 -> [_ w412]
          frame False {
          }
          frame True {
            n207 = Subtract(x=180.0, y=w412) -> (x-y=w414:dbl)
            n208 = Add(x=w414, y=w413) -> (x+y=w410:dbl)
            n209 = Add(x=w417, y=w418) -> (x+y=w416:dbl)
            n210 = Less?(x=w410, y=7.0) -> (x < y?=w419:bool)
            n211 = Select(t=w416, s=w419, f=w418) -> (s? t:f=w415:dbl)
          }
        }
        n212 = call <vilib>:"CTRE_Phoenix_MotorControl_Set.vi"("Output"=w385, "Control Mode"=w393, "PhoenixMotorControlDevRef"=w395) -> ()  [unwired: 7 in, 2 out]
        n213 = call <vilib>:"CTRE_Phoenix_MotorControl_Set.vi"("Output"=w392, "Control Mode"=w393, "PhoenixMotorControlDevRef"=w394) -> ()  [unwired: 7 in, 2 out]
        n214 = call <vilib>:"CTRE_Phoenix_MotorControl_Set.vi"("Output"=w386, "Control Mode"=w393, "PhoenixMotorControlDevRef"=w396) -> ()  [unwired: 7 in, 2 out]
        n215 = call <vilib>:"CTRE_Phoenix_MotorControl_Set.vi"("Output"=w390, "Control Mode"=w393, "PhoenixMotorControlDevRef"=w391) -> ()  [unwired: 7 in, 2 out]
      }
      frame "Move arm to position" {
        w437 = T22 7 items=["PercentOutput"=0, "Position"=1, "Velocity"=2, "Current"=3, "Follower"=5, "MotionProfile"=6, "MotionMagic"=7, "MotionProfileArc"=10, "Disabled"=15] ("Control Mode")
        w440 = 100.0  # Wait ms
        n216 = Index Array(array=w425) -> (element #1=w421:bool, element #2=w422:bool, element #3=w423:bool, element #4=w424:bool)  [unwired: 4 in]
        n217 = call "AngleToWristEncoder.vi"("angle(deg)"=w426) -> ("encoderPulses"=w433:i32)  [unwired: 10 in]
        n218 = call "AngleToTurretEncoder.vi"("angle(deg)"=w429) -> ("encoderPulses"=w434:i32)  [unwired: 10 in]
        n219 = call "AngleToShoulderEncoder.vi"("angle(deg)"=w428) -> ("encoderPulses"=w431:i32)  [unwired: 10 in]
        n220 = call "AngleToElbowEncoder.vi"("angle(deg)"=w427) -> ("encoderPulses"=w432:i32)  [unwired: 10 in]
        n221 = case shown="True" w421 {
          tunnel: w437 -> [_ w452]
          tunnel: w436 -> [_ w451]
          tunnel: w434 -> [_ w450]
          frame False {
          }
          frame True {
            n222 = call <vilib>:"CTRE_Phoenix_MotorControl_Set.vi"("Output"=w450, "Control Mode"=w452, "PhoenixMotorControlDevRef"=w451) -> ()  [unwired: 7 in, 2 out]
          }
        }
        n223 = case shown="True" w422 {
          tunnel: w439 -> [_ w449]
          tunnel: w437 -> [_ w448]
          tunnel: w431 -> [_ w447]
          frame False {
          }
          frame True {
            n224 = call <vilib>:"CTRE_Phoenix_MotorControl_Set.vi"("Output"=w447, "Control Mode"=w448, "PhoenixMotorControlDevRef"=w449) -> ()  [unwired: 7 in, 2 out]
          }
        }
        n225 = case shown="True" w423 {
          tunnel: w437 -> [_ w446]
          tunnel: w435 -> [_ w445]
          tunnel: w432 -> [_ w444]
          frame False {
          }
          frame True {
            n226 = call <vilib>:"CTRE_Phoenix_MotorControl_Set.vi"("Output"=w444, "Control Mode"=w446, "PhoenixMotorControlDevRef"=w445) -> ()  [unwired: 7 in, 2 out]
          }
        }
        n227 = case shown="True" w424 {
          tunnel: w438 -> [_ w443]
          tunnel: w437 -> [_ w442]
          tunnel: w433 -> [_ w441]
          frame False {
          }
          frame True {
            n228 = call <vilib>:"CTRE_Phoenix_MotorControl_Set.vi"("Output"=w441, "Control Mode"=w442, "PhoenixMotorControlDevRef"=w443) -> ()  [unwired: 7 in, 2 out]
          }
        }
      }
      frame "Hold Encoder Counts" {
        w459 = 100.0  # Wait ms
        n229 = case shown="True" w453 {
          tunnel: w457 -> [_ w470]
          tunnel: w456 -> [_ w468]
          tunnel: w455 -> [_ w465]
          tunnel: w454 -> [_ w462]
          frame False {
          }
          frame True {
            w472 = T22 7 items=["PercentOutput"=0, "Position"=1, "Velocity"=2, "Current"=3, "Follower"=5, "MotionProfile"=6, "MotionMagic"=7, "MotionProfileArc"=10, "Disabled"=15] ("Control Mode")
            n230 = call-poly <vilib>:"CTRE_Phoenix_MotorController_Get_Enhanced.vi"("PhoenixMotorControlDevRef"=w470) -> ("PhoenixMotorControlDevRef"=w471:T12, "Position (Raw Sensor Units)"=w469:i32)  [unwired: 11 in, 2 out]
            n231 = call-poly <vilib>:"CTRE_Phoenix_MotorController_Get_Enhanced.vi"("PhoenixMotorControlDevRef"=w468) -> ("PhoenixMotorControlDevRef"=w467:T12, "Position (Raw Sensor Units)"=w466:i32)  [unwired: 11 in, 2 out]
            n232 = call-poly <vilib>:"CTRE_Phoenix_MotorController_Get_Enhanced.vi"("PhoenixMotorControlDevRef"=w462) -> ("PhoenixMotorControlDevRef"=w461:T12, "Position (Raw Sensor Units)"=w460:i32)  [unwired: 11 in, 2 out]
            n233 = call-poly <vilib>:"CTRE_Phoenix_MotorController_Get_Enhanced.vi"("PhoenixMotorControlDevRef"=w465) -> ("PhoenixMotorControlDevRef"=w464:T12, "Position (Raw Sensor Units)"=w463:i32)  [unwired: 11 in, 2 out]
            n234 = call <vilib>:"CTRE_Phoenix_MotorControl_Set.vi"("Output"=w463, "Control Mode"=w472, "PhoenixMotorControlDevRef"=w464) -> ()  [unwired: 7 in, 2 out]
            n235 = call <vilib>:"CTRE_Phoenix_MotorControl_Set.vi"("Output"=w460, "Control Mode"=w472, "PhoenixMotorControlDevRef"=w461) -> ()  [unwired: 7 in, 2 out]
            n236 = call <vilib>:"CTRE_Phoenix_MotorControl_Set.vi"("Output"=w466, "Control Mode"=w472, "PhoenixMotorControlDevRef"=w467) -> ()  [unwired: 7 in, 2 out]
            n237 = call <vilib>:"CTRE_Phoenix_MotorControl_Set.vi"("Output"=w469, "Control Mode"=w472, "PhoenixMotorControlDevRef"=w471) -> ()  [unwired: 7 in, 2 out]
          }
        }
      }
      frame "Reserve", Default {
        w474 = -1.0  # Infinite
        # "If loop needs to poll sensors or other\nvalues, use a timeout value. -1 waits for\nnext command to be sent."
      }
      frame "Read Current" {
      }
      frame "Reset Encoders" {
        w479 = 0 ("New Sensor Position")
        n238 = call <vilib>:"CTRE_Phoenix_MotorControl_SetSelectedSensorPosition.vi"("New Sensor Position"=w479, "PhoenixMotorControlDevRef"=w483) -> ()  [unwired: 8 in, 2 out]
        n239 = call <vilib>:"CTRE_Phoenix_MotorControl_SetSelectedSensorPosition.vi"("New Sensor Position"=w479, "PhoenixMotorControlDevRef"=w480) -> ()  [unwired: 8 in, 2 out]
        n240 = call <vilib>:"CTRE_Phoenix_MotorControl_SetSelectedSensorPosition.vi"("New Sensor Position"=w479, "PhoenixMotorControlDevRef"=w481) -> ()  [unwired: 8 in, 2 out]
        n241 = call <vilib>:"CTRE_Phoenix_MotorControl_SetSelectedSensorPosition.vi"("New Sensor Position"=w479, "PhoenixMotorControlDevRef"=w482) -> ()  [unwired: 8 in, 2 out]
      }
      frame "Reset Turret" {
        n242 = call <vilib>:"CTRE_Phoenix_MotorControl_SetSelectedSensorPosition.vi"("New Sensor Position"=0, "PhoenixMotorControlDevRef"=w486) -> ()  [unwired: 8 in, 2 out]
      }
      frame "Reset Shoulder" {
        n243 = call <vilib>:"CTRE_Phoenix_MotorControl_SetSelectedSensorPosition.vi"("New Sensor Position"=0, "PhoenixMotorControlDevRef"=w490) -> ()  [unwired: 8 in, 2 out]
      }
      frame "Reset Elbow" {
        n244 = call <vilib>:"CTRE_Phoenix_MotorControl_SetSelectedSensorPosition.vi"("New Sensor Position"=0, "PhoenixMotorControlDevRef"=w494) -> ()  [unwired: 8 in, 2 out]
      }
      frame "Reset Wrist" {
        n245 = call <vilib>:"CTRE_Phoenix_MotorControl_SetSelectedSensorPosition.vi"("New Sensor Position"=0, "PhoenixMotorControlDevRef"=w498) -> ()  [unwired: 8 in, 2 out]
      }
    }
    n246 = call "Arm Check for New Command.vi"("Current Command"=w355, "Wait time (ms)"=w360, "Finished?"=w361) -> ("Completion"=w356:T7, "Subsystem Name"=w357:string, "Current Command"=w358:T4, "Initial Trace String"=w359:string, "NextCommand"=w362:T19)  [unwired: 4 in]
    n247 = case shown="\"Successful\", \"Aborted\"" w356 {
      selector: w356 -> [_ w377]
      tunnel: w359 -> [_ w373]
      tunnel: w358 -> [_ w374]
      tunnel: w357 -> [_ w370]
      frame "Incomplete", Default {
        # "Continuing current command"
      }
      frame "Successful", "Aborted" {
        # "Report and setup for next command"
        n248 = Unbundle By Name(w374) -> ("Turret Setpoint"=w376:dbl, "Shoulder Setpoint"=w371:dbl)
        n249 = Format Into String(format string="S %.1f, D %f", initial string=w373, w376, w371) -> (resulting string=w372:string)  [unwired: 1 in, 1 out]
        "Current\nCmd" <- w372
        n250 = call <vilib>:"Trace Results.vi"("Status of previous command"=w377, "Description"=w372, "Subsystem"=w370) -> ()  [unwired: 9 in]
      }
    }
    n251 = disable-structure shown="Disabled" {
      frame Disabled {
        # "Publish"
        n252 = call-poly <vilib>:"NT Write Value.vi"() -> ()  [unwired: 11 in, 1 out]
      }
      frame Enabled {
      }
    }
  }
